vi "启动参数设置.vi"() -> ()   [LabVIEW 2016, in "斯坦道氟化物.lvlib"]
panel:
  in  "CODMn":bool
  in  "氟化物":bool
  in  "关闭":bool
  in  "保存":bool
  out "启动队列名称":cluster{"String":string, "Value":u16}[](array[cluster])
  out "启动参数":string
  in  "CODcr":bool
  in  "硫化物":bool
  in  "硅酸盐":bool
  in  "亚硝氮":bool
  in  "硝氮":bool
  in  "磷酸盐":bool
  in  "氨氮":bool
  in  "总氮":bool
  in  "总磷":bool
  # "请选择要启动的参数"
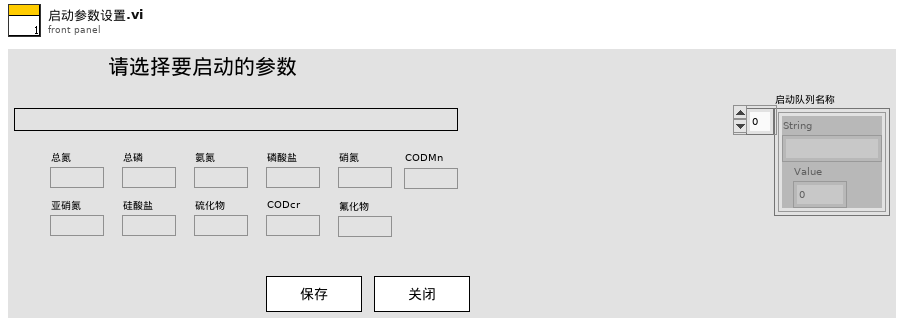
[diagram p1: front panel]
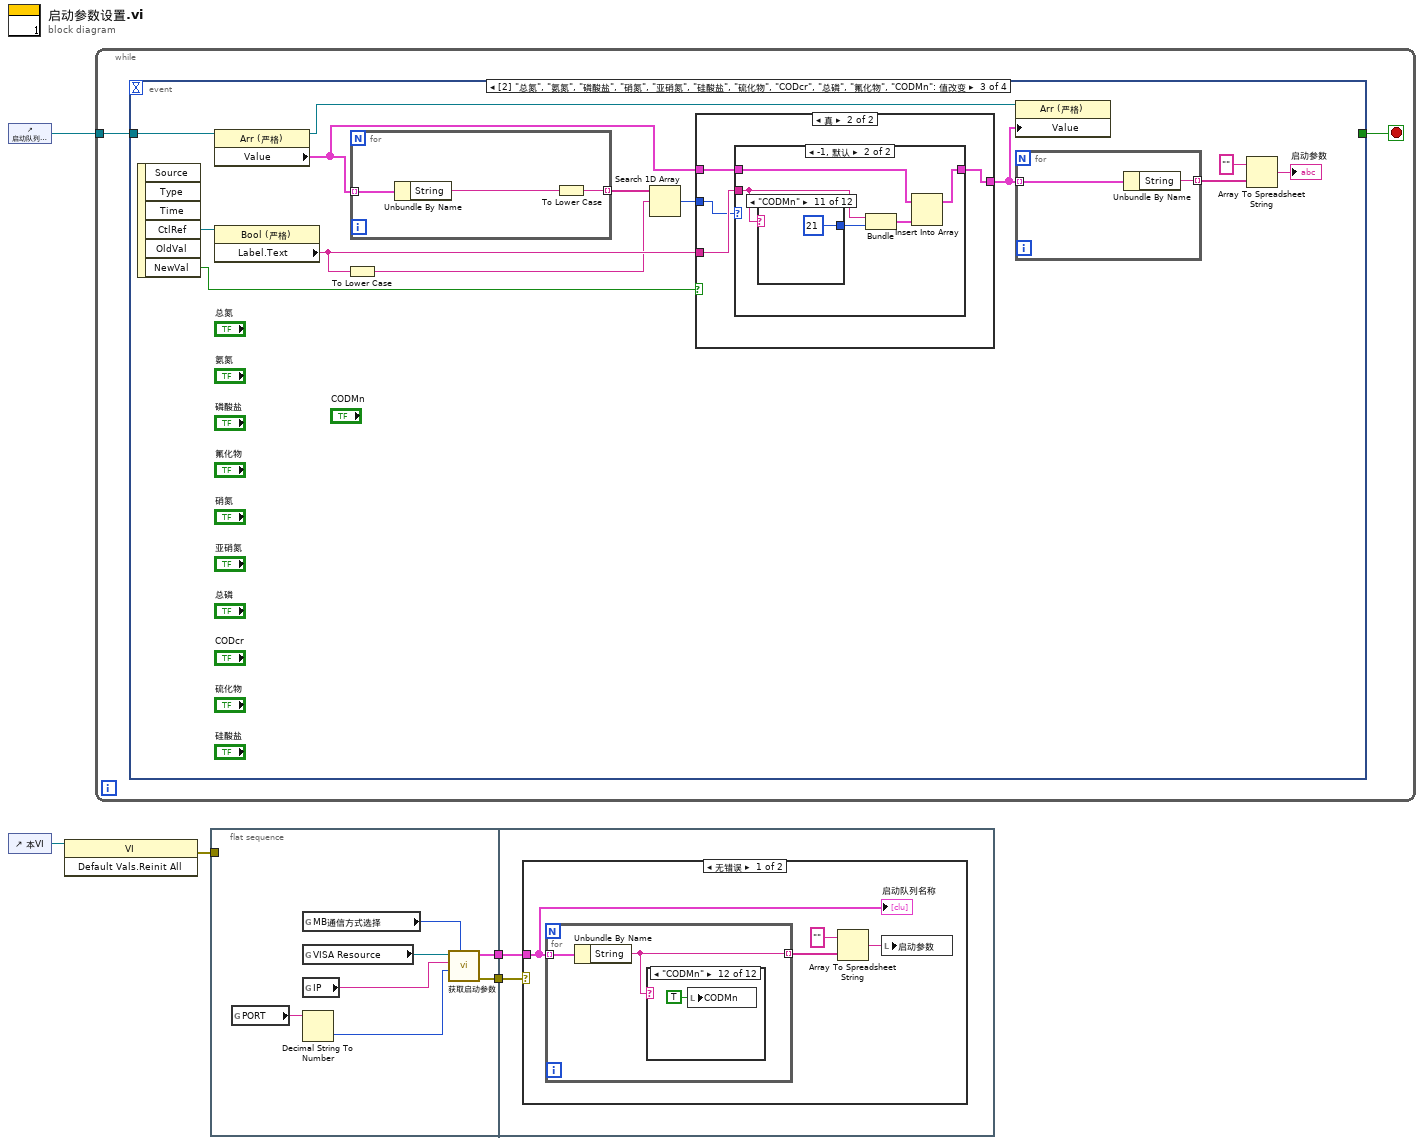
[diagram p0: block diagram]
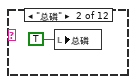
[diagram p3: hidden frame]
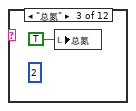
[diagram p4: hidden frame]
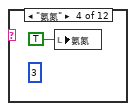
[diagram p5: hidden frame]
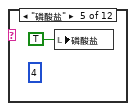
[diagram p6: hidden frame]
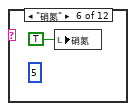
[diagram p7: hidden frame]
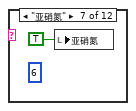
[diagram p8: hidden frame]
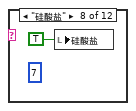
[diagram p9: hidden frame]
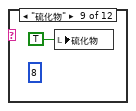
[diagram p10: hidden frame]
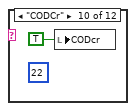
[diagram p11: hidden frame]
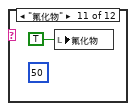
[diagram p12: hidden frame]
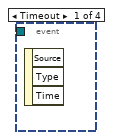
[diagram p14: hidden frame]
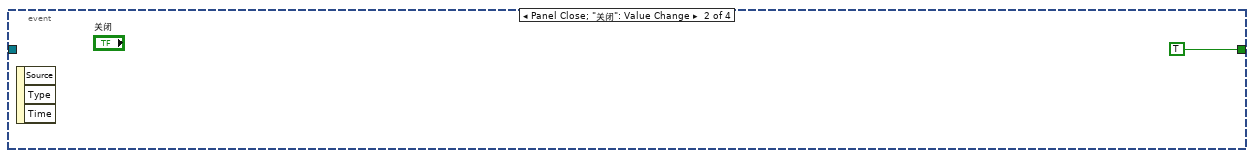
[diagram p15: hidden frame]
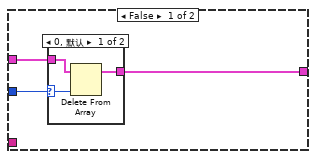
[diagram p16: hidden frame]
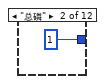
[diagram p20: hidden frame]
diagram:
  n1 = control-ref of="启动队列名称"() -> (w5:refnum<vi>)
  n2 = control-ref of="本VI"() -> (w4:refnum<vi>)
  n3 = invoke class="VI" method="Default Vals.Reinit All"(reference=w4) -> (error out=w3:errorcluster)  [unwired: 2 in, 2 out]
  n4 = while {
    tunnel: w5 -> [w6]
    stop <- w7 stop-if-true
    n5 = event shown="[2] \"总氮\", \"氨氮\", \"磷酸盐\", \"硝氮\", \"亚硝氮\", \"硅酸盐\", \"硫化物\", \"CODcr\", \"总磷\", \"氟化物\", \"CODMn\": 值改变" {
      selector: _ -> [_ _ _ _]
      dyn-events: _ -> [_ _ _ _]
      timeout: _ -> [_ _ _ _]
      tunnel: [_ TRUE _ _] -> w7
      tunnel: w6 -> [_ _ w13 w61]
      event Timeout {
        n6 = event-data() -> ()  [unwired: 1 in, 3 out]
      }
      event Panel Close; "关闭": Value Change {
        n7 = event-data() -> ()  [unwired: 1 in, 3 out]
      }
      event "总氮", "氨氮", "磷酸盐", "硝氮", "亚硝氮", "硅酸盐", "硫化物", "CODcr", "总磷", "氟化物", "CODMn": Value Change {
        n8 = event-data() -> ("CtlRef"=w21:refnum<vi>, "NewVal"=w20:bool)  [unwired: 1 in, 4 out]
        n9 = property class="Arr (严格)"(reference=w13) -> (reference out=w11:refnum<vi>, "Value"=w12:cluster{"String":string, "Value":u16}[])  [unwired: 1 in, 1 out]
        n10 = property class="Bool (严格)"(reference=w21) -> ("Label.Text"=w18:string)  [unwired: 1 in, 2 out]
        n11 = To Lower Case(string=w18) -> (all lower case string=w9:string)
        n12 = for {
          tunnel: w12 -> [w26] mode=indexing
          tunnel: [w24] -> w19 mode=indexing
          n13 = Unbundle By Name(w26) -> ("String"=w25:string)
          n14 = To Lower Case(string=w25) -> (all lower case string=w24:string)
        }
        n15 = Search 1D Array(1D array=w19, element=w9) -> (index of element=w17:i32)  [unwired: 1 in]
        n16 = case shown="真" w20 {
          tunnel: w18 -> [_ w36]
          tunnel: w12 -> [w28 w37]
          tunnel: w17 -> [w29 w35]
          tunnel: [w27 w34] -> w10
          frame False {
            n17 = case shown="0, 默认" w29 {
              selector: w29 -> [w31 _]
              tunnel: w28 -> [w32 w33]
              tunnel: [w30 w33] -> w27
              frame 0, Default {
                n18 = Delete From Array(array=w32, index=w31) -> (array with subset deleted=w30:cluster{"String":string, "Value":u16}[])  [unwired: 1 in, 1 out]
              }
              frame -1 {
              }
            }
          }
          frame True {
            n19 = case shown="-1, 默认" w35 {
              tunnel: w37 -> [w38 w43]
              tunnel: w36 -> [_ w42]
              tunnel: [w38 w39] -> w34
              frame 0 {
              }
              frame -1, Default {
                n20 = case shown="\"CODMn\"" w42 {
                  tunnel: [_ 1 2 3 4 5 6 7 8 22 21 50] -> w41
                  frame Default {
                  }
                  frame "总磷" {
                  }
                  frame "总氮" {
                  }
                  frame "氨氮" {
                  }
                  frame "磷酸盐" {
                  }
                  frame "硝氮" {
                  }
                  frame "亚硝氮" {
                  }
                  frame "硅酸盐" {
                  }
                  frame "硫化物" {
                  }
                  frame "CODCr" {
                  }
                  frame "CODMn" {
                  }
                  frame "氟化物" {
                  }
                }
                n21 = Bundle("Label.Text"=w42, w41) -> (w40:cluster{"Label.Text":string, i32})  [unwired: 1 in]
                n22 = Insert Into Array(array=w43, new element=w40) -> (w39:cluster{"String":string, "Value":u16}[])  [unwired: 1 in]
              }
            }
          }
        }
        n23 = property class="Arr (严格)"(reference=w11, "Value"=w10) -> ()  [unwired: 1 in, 2 out]
        n24 = for {
          tunnel: w10 -> [w23] mode=indexing
          tunnel: [w22] -> w16 mode=indexing
          n25 = Unbundle By Name(w23) -> ("String"=w22:string)
        }
        n26 = Array To Spreadsheet String(array=w16, 3:"" ("格式字符串")) -> (spreadsheet string=→"启动参数":string)  [unwired: 1 in]
      }
      event "保存": Value Change {
        n27 = event-data() -> ()  [unwired: 1 in, 6 out]
        n28 = global read "总磷总氮断电保存全局变量.vi" "PORT"() -> (w57:string)
        n29 = property class="Arr (严格)"(reference=w61) -> ("Value"=w55:cluster{"String":string, "Value":u16}[])  [unwired: 1 in, 2 out]
        n30 = Decimal String To Number(string=w57) -> (number=w56:i32)  [unwired: 2 in, 1 out]
        n31 = flat-sequence {
          tunnel: w55 -> [w62]
          frame #0 {
            n32 = global write "model config var.vi" "启动队列名称"(w62) -> ()
          }
          frame #1 {
            n33 = call "模块配置写入.vi"() -> ()  [unwired: 11 in, 1 out]
          }
        }
        n34 = global read "总磷总氮断电保存全局变量.vi" "MB通信方式选择"() -> (w60:enum16{"串口", "TCP"})
        n35 = global read "总磷总氮断电保存全局变量.vi" "VISA Resource"() -> (w59:refnum<visa-resource-name>)
        n36 = global read "总磷总氮断电保存全局变量.vi" "IP"() -> (w58:string)
        n37 = call "设置启动参数.vi"("数组"=w55, "MB通信方式选择"=w60, "Port (502)"=w56, "IP Address"=w58, "VISA Resource"=w59) -> ()  [unwired: 6 in, 1 out]
      }
    }
  }
  n38 = flat-sequence {
    tunnel: w3 -> [_]
    tunnel: [w64] -> w2
    tunnel: [w63] -> w1
    tunnel: w2 -> [w71]
    tunnel: w1 -> [w70]
    frame #0 {
      n39 = global read "总磷总氮断电保存全局变量.vi" "PORT"() -> (w65:string)
      n40 = global read "总磷总氮断电保存全局变量.vi" "MB通信方式选择"() -> (w66:enum16{"串口", "TCP"})
      n41 = global read "总磷总氮断电保存全局变量.vi" "VISA Resource"() -> (w67:refnum<visa-resource-name>)
      n42 = global read "总磷总氮断电保存全局变量.vi" "IP"() -> (w68:string)
      n43 = Decimal String To Number(string=w65) -> (number=w69:i32)  [unwired: 2 in, 1 out]
      n44 = call "获取启动参数.vi"("MB通信方式选择"=w66, "Port (502)"=w69, "IP Address"=w68, "VISA Resource"=w67) -> ("error out"=w63:errorcluster, "数组"=w64:cluster{"String":string, "Value":u16}[])  [unwired: 6 in]
    }
    frame #1 {
      n45 = case shown="无错误" w70 {
        tunnel: w71 -> [w72 _]
        frame No Error {
          n46 = for {
            tunnel: w72 -> [w77] mode=indexing
            tunnel: [w76] -> w74 mode=indexing
            n47 = Unbundle By Name(w77) -> ("String"=w76:string)
            n48 = case shown="\"CODMn\"" w76 {
              frame Default {
              }
              frame "总磷" {
                n49 = local write "总磷"(TRUE ("总磷")) -> ()
              }
              frame "总氮" {
                (unwired) 2
                n50 = local write "总氮"(TRUE ("总磷")) -> ()
              }
              frame "氨氮" {
                (unwired) 3
                n51 = local write "氨氮"(TRUE ("总磷")) -> ()
              }
              frame "磷酸盐" {
                (unwired) 4
                n52 = local write "磷酸盐"(TRUE ("总磷")) -> ()
              }
              frame "硝氮" {
                (unwired) 5
                n53 = local write "硝氮"(TRUE ("总磷")) -> ()
              }
              frame "亚硝氮" {
                (unwired) 6
                n54 = local write "亚硝氮"(TRUE ("总磷")) -> ()
              }
              frame "硅酸盐" {
                (unwired) 7
                n55 = local write "硅酸盐"(TRUE ("总磷")) -> ()
              }
              frame "硫化物" {
                (unwired) 8
                n56 = local write "硫化物"(TRUE ("总磷")) -> ()
              }
              frame "CODCr" {
                (unwired) 22
                n57 = local write "CODcr"(TRUE ("总磷")) -> ()
              }
              frame "氟化物" {
                (unwired) 50
                n58 = local write "氟化物"(TRUE ("总磷")) -> ()
              }
              frame "CODMn" {
                n59 = local write "CODMn"(TRUE ("总磷")) -> ()
              }
            }
          }
          n60 = Array To Spreadsheet String(array=w74, 3:"" ("格式字符串")) -> (spreadsheet string=w73:string)  [unwired: 1 in]
          n61 = local write "启动参数"(w73) -> ()
          "启动队列名称" <- w72
        }
        frame Error {
        }
      }
    }
  }
